vi "Version3.0.vi"() -> ()   [LabVIEW 2012]
uses:
  <vilib>/Instr/_visa.llb/VISA Configure Serial Port (Instr).vi
  Function_Set/Debug/Function_Set.dll
panel:
  in  "选项卡控件":enum32{"Note", "AVT CCD", "Vacuum REC", "..."}(tab)
  in  "Double:":dbl
  in  "String:":string
  in  "Other:":string
  in  "Save This Shot":bool
  out "Shots:":i32
  in  "Save This Notes":bool
  in  "Other Notes:":string
  out "Shot's situation:":string
  out "Shots: 2":i32
  out "Notes:":string
  in  "查询":bool
  in  "Options":u16(ring) caption="Choose File:"
  in  "Initial Folder Path:":path
  in  "Your Own:":u16(ring) items=["2, 10000, 3, 1", "2, 10000, 4, 1"]
  in  "FrameStartTriggerMode":T1(ring)
  in  "AcquisitionMode":T2(ring)
  in  "ExposureMode":T3(ring)
  in  "AVT SDK Demon":bool
  out "CCD ID":string
  out "ExposureMode":string
  out "ExposureValue":u32
  out "AcquisitionMode":string
  out "FrameStartTriggerMode":string
  in  "ExposureValue":u32
  in  "CameraStart":bool
  in  "CameraStop":bool
  in  "CameraSet":bool
  in  "CameraGet":bool
  in  "CameraSetAll":bool
  in  "path to JPEG file":path caption="Path of the Pic"
  out "new picture":picture caption="Pic"
  in  "端口选择":refnum<visa-resource-name>="COM1"
  in  "baud rate":u32=9600
  in  "data bits":u16=8
  in  "stop bits":u16(ring)=10 items=["1.0"=10, "1.5"=15, "2.0"=20]
  in  "flow control":u16(ring) items=["None"=0, "XON/XOFF"=1, "RTS/CTS"=2, "DTR/DSR"=4]
  in  "timeout":u32=10
  in  "RS485地址":string="12"
  in  "读取间隔(s)":dbl=1.0 caption="Delay Time (s)"
  in  "数据文件夹":string="data"
  in  "记录说明":string="test"
  out "数据路径":path
  in  "parity (0:none)":enum16{"None", "Odd", "Even", "Mark", "Space"}(ring)
  in  "记录所有读取数据?":bool
  out "已记录数据点":u32 caption="recorded number"
  in  "stop":bool
  out "电离规图表":dbl(graph)
  out "电阻规图表":dbl(graph)
  out "已读取数据点":i32
  out "预定耗时":dbl
  out "实际耗时":dbl
  in  "临界压强(Pa)":dbl=8.0
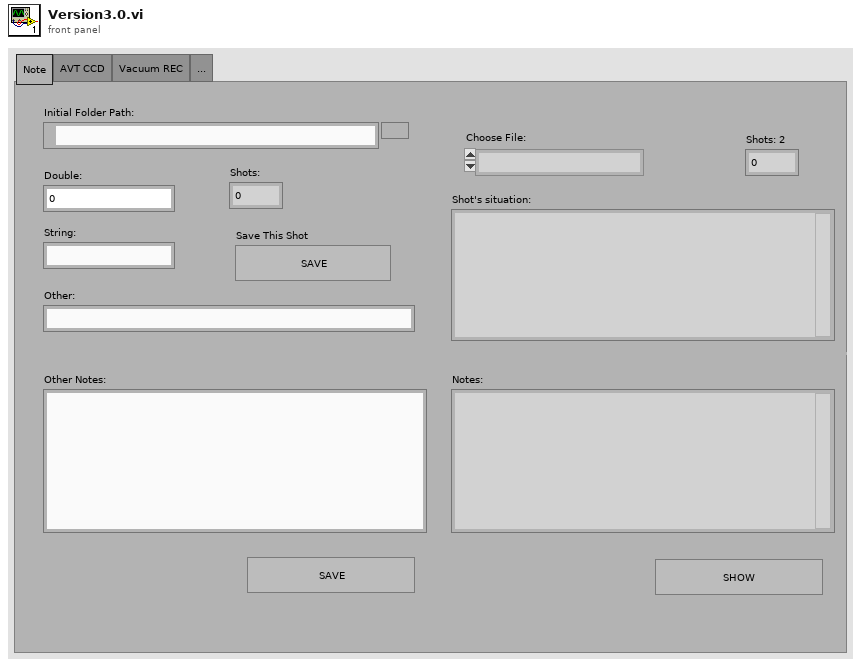
[diagram p1: front panel]
types:
  T1 = enum16{"默认", "Freerun", "SyncIn1", "SyncIn2", "FixedRate", "Software"}
  T2 = enum16{"默认", "Continuous", "SingleFrame", "MultiFrame", "Recorder"}
  T3 = enum16{"默认", "Manual", "Auto", "AutoOnce", "External"}
  T4 = cluster{"Resister":dbl, "Ionization":dbl, "time":string, "Ionization":dbl, "Ionization":dbl, u32, i32}
  T5 = enum32{"Record", "Instrument 1", "Instrument 2", "..."}
  T6 = enum16{"open", "replace", "create", "open or create", "replace or create", "replace or create with confirmation"}
  T7 = typedef "imagedata.ctl" = cluster{"image type":i32, "image depth":i32, "image":u8[], "mask":u8[], "colors":u32[], "Rectangle":cluster{"left":i16, "top":i16, "right":i16, "bottom":i16}}
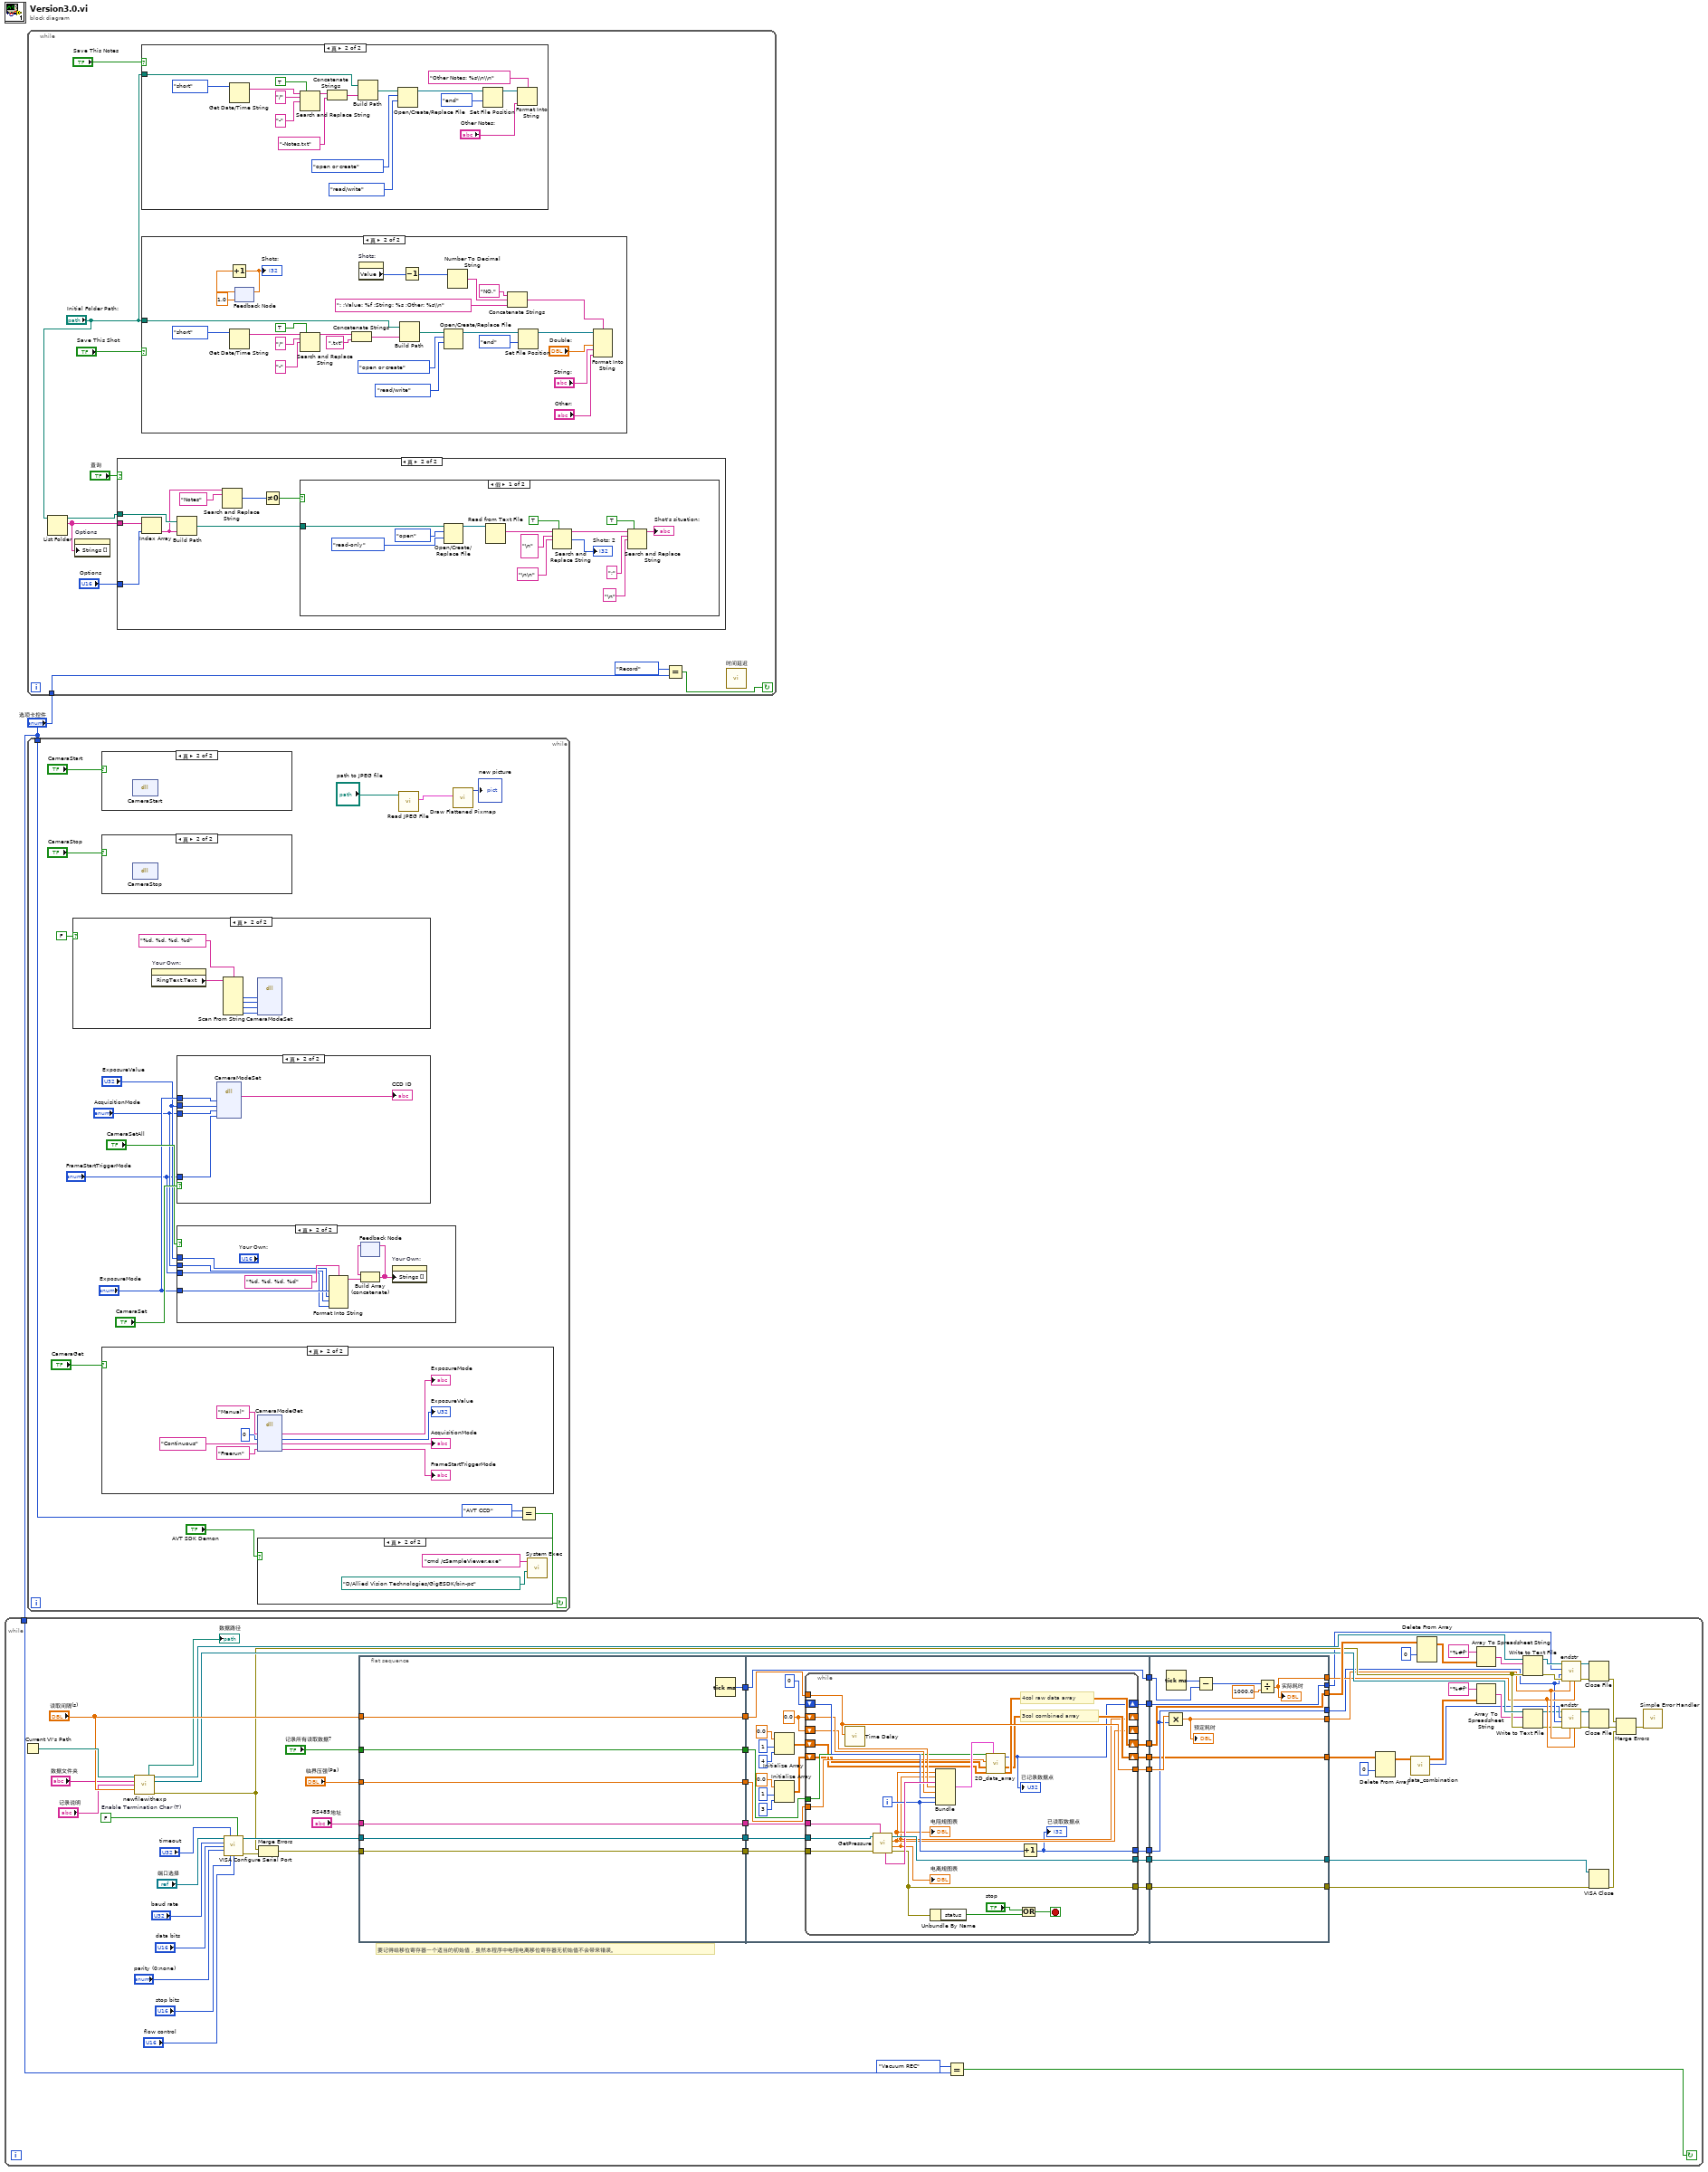
[diagram p0: block diagram]
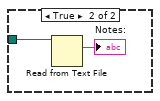
[diagram p10: hidden frame]
diagram:
  n1 = while {
    tunnel: "选项卡控件" -> [w3]
    stop <- w4 continue-if-true
    w54 = FALSE  # Enable Termination Char (T)
    # "要记得给移位寄存器一个适当的初始值，虽然本程序中电阻电离移位寄存器无初始值不会带来错误。"
    n2 = Current VI's Path() -> (path=w46:path)
    n3 = call "newfilewithexp.vi"("路径"=w46, "数据文件夹"="数据文件夹", "记录说明"="记录说明", "读取间隔(s)"="读取间隔(s)") -> ("数据路径"=→"数据路径":path, "refnum out for 4column"=w25:refnum<file>, "refnum out for 3column"=w23:refnum<file>, "error out"=w22:errorcluster)  [unwired: 1 in, 7 out]
    n4 = call-poly "VISA Configure Serial Port"("VISA resource name"="端口选择", "timeout (10sec)"="timeout", "Enable Termination\nChar (T)"=w54, "baud rate (9600)"="baud rate", "data bits (8)"="data bits", "parity (0:none)"="parity (0:none)", "stop bits (10: 1 bit)"="stop bits", "flow control (0:none)"="flow control") -> ("VISA resource name out"=w51:refnum<visa-resource-name>, "error out"=w26:errorcluster)  [unwired: 1 in, 5 out]
    n5 = Merge Errors(w22, w26) -> (w34:errorcluster)
    n6 = flat-sequence {
      tunnel: "RS485地址" -> [w74]
      tunnel: "读取间隔(s)" -> [w75]
      tunnel: "记录所有读取数据?" -> [w76]
      tunnel: w34 -> [w77]
      tunnel: w51 -> [w78]
      tunnel: [w78] -> w71
      tunnel: [w77] -> w70
      tunnel: [w76] -> w69
      tunnel: [w75] -> w68
      tunnel: [w74] -> w67
      tunnel: [w73] -> w66
      tunnel: "临界压强(Pa)" -> [w72]
      tunnel: [w72] -> w65
      tunnel: [w100] -> w64
      tunnel: [w79] -> w63
      tunnel: w71 -> [w102]
      tunnel: w70 -> [w101]
      tunnel: w69 -> [w98]
      tunnel: w68 -> [w97]
      tunnel: w67 -> [w96]
      tunnel: [w95] -> w62
      tunnel: w66 -> [w95]
      tunnel: [w94] -> w61
      tunnel: [w93] -> w60
      tunnel: w65 -> [w92]
      tunnel: [w91] -> w59
      tunnel: [w85] -> w58
      tunnel: [w80] -> w57
      tunnel: [w139] -> w49
      tunnel: [w140] -> w50
      tunnel: w64 -> [w140]
      tunnel: w63 -> [w139]
      tunnel: w62 -> [w137]
      tunnel: w61 -> [w131]
      tunnel: w60 -> [w134]
      tunnel: w59 -> [w132]
      tunnel: w58 -> [w133]
      tunnel: [w133] -> w39
      tunnel: [w132] -> w18
      tunnel: [w131] -> w17
      tunnel: [w130] -> w20
      tunnel: [w129] -> w19
      tunnel: w57 -> [w128]
      tunnel: [w128] -> w33
      frame #0 {
        n7 = Tick Count (ms)() -> (millisecond timer value=w73:u32)
      }
      frame #1 {
        w90 = 0.0 ("Ionization")
        n8 = Initialize Array(0.0 ("element"), 1 ("dimension size"), 4 ("dimension size")) -> (w88:dbl[][])
        n9 = Initialize Array(0.0 ("element"), 1 ("dimension size"), 3 ("dimension size")) -> (w81:dbl[][])
        n10 = while {
          tunnel: w102 -> [w127]
          tunnel: w101 -> [w126]
          tunnel: w96 -> [w123]
          tunnel: [w109] -> w100
          tunnel: [w124] -> w79
          shift-right: [w110] -> w91
          shift-left: u32 0 -> [w120]
          shift-right: [w104] -> _
          shift-left: w90 -> [w119]
          tunnel: w97 -> [w125]
          tunnel: w98 -> [w116]
          tunnel: [w103] -> w94
          tunnel: [w125] -> w93
          shift-right: [w105] -> _
          shift-left: w90 -> [w118]
          tunnel: w92 -> [w115]
          shift-right: [w113] -> w85
          shift-left: w88 -> [w114]
          shift-right: [w111] -> w80
          shift-left: w81 -> [w112]
          i -> [w121]
          stop <- w106 stop-if-true
          # "4col raw data array"
          # "3col combined array"
          n11 = call "Time Delay"("Delay Time (s)"=w125) -> ()  [unwired: 1 in, 10 out]
          n12 = call "GetPressure.vi"("Address of RS485"=w123, "error in (no error)"=w126, "VISA resource name"=w127) -> ("error out"=w109:errorcluster, "Ionization"=w104:dbl, "Resister"=w105:dbl, "VISA resource name out"=w124:refnum<visa-resource-name>, "time"=w122:string)  [unwired: 1 in, 3 out]
          "电阻规图表" <- w105
          "电离规图表" <- w104
          n13 = Unbundle By Name(w109) -> ("status"=w107:bool)
          n14 = Bundle("Resister"=w105, "Ionization"=w104, "time"=w122, "Ionization"=w118, "Ionization"=w119, w120, w121) -> (w117:T4)  [unwired: 1 out]
          n15 = call "2D_data_array.vi"("input cluster"=w117, "input 4column array"=w114, "input combined 3column array"=w112, "critical pressure"=w115, "record all data points?"=w116) -> ("output 4column array"=w113:dbl[][], "output combined 3column array"=w111:dbl[][], "recorded number out"=w110:u32)  [unwired: 4 out]
          "已记录数据点" <- w110
          n16 = Or(x="stop", y=w107) -> (x .or. y?=w106:bool)
          n17 = Increment(x=w121) -> (x+1=w103:i32)
          "已读取数据点" <- w103
        }
      }
      frame #2 {
        n18 = Multiply(x=w134, y=w131) -> (x*y=w130:dbl)
        "预定耗时" <- w130
        n19 = Tick Count (ms)() -> (millisecond timer value=w138:u32)
        n20 = Subtract(x=w138, y=w137) -> (x-y=w136:u32)
        n21 = Divide(x=w136, y=1000.0) -> (x/y=w129:dbl)
        "实际耗时" <- w129
      }
    }
    n22 = Equal?(x=enum32{"Note", "AVT CCD", "Vacuum REC", "..."}."Vacuum REC", y=w3) -> (x = y?=w4:bool)
    n23 = Delete From Array(array=w33, index (row)=0) -> (array with subset deleted=w30:dbl[][])  [unwired: 2 in, 1 out]
    n24 = call "data_combination.vi"("input combined data array"=w30) -> ("recorded combined data number"=w16:i32, "output combined data array"=w27:dbl[][])  [unwired: 9 out]
    n25 = Delete From Array(array=w39, index (row)=0) -> (array with subset deleted=w40:dbl[][])  [unwired: 2 in, 1 out]
    n26 = Array To Spreadsheet String(array=w40, 3:"%#f" ("format string")) -> (spreadsheet string=w24:string)  [unwired: 1 out]
    n27 = Array To Spreadsheet String(array=w27, 3:"%#f" ("format string")) -> (spreadsheet string=w21:string)  [unwired: 1 out]
    n28 = Write to Text File(file (use dialog)=w25, text=w24, error in=w22) -> (refnum out=w36:refnum<file>, error out=w35:errorcluster)  [unwired: 2 out]
    n29 = Write to Text File(file (use dialog)=w23, text=w21, error in=w22) -> (refnum out=w15:refnum<file>, error out=w14:errorcluster)  [unwired: 2 out]
    n30 = call "endstr.vi"("实际耗时"=w19, "预定耗时"=w20, "error in"=w35, "已读取数据点"=w17, "已记录数据点"=w18, "refnum in"=w36) -> ("error out"=w38:errorcluster, "refnum out"=w37:refnum<file>)  [unwired: 4 out]
    n31 = call "endstr.vi"("实际耗时"=w19, "预定耗时"=w20, "error in"=w14, "已读取数据点"=w17, "已记录数据点"=w16, "refnum in"=w15) -> ("error out"=w28:errorcluster, "refnum out"=w29:refnum<file>)  [unwired: 4 out]
    n32 = Close File(refnum=w37, error in=w38) -> (error out=w10:errorcluster)  [unwired: 1 out]
    n33 = Close File(refnum=w29, error in=w28) -> (error out=w11:errorcluster)  [unwired: 1 out]
    n34 = VISA Close(VISA resource name=w49, error in (no error)=w50) -> (error out=w12:errorcluster)
    n35 = Merge Errors(w10, w11, w12) -> (w13:errorcluster)
    n36 = call <vilib>:"Simple Error Handler.vi"("error in (no error)"=w13) -> ()  [unwired: 1 in, 8 out]
  }
  n37 = while {
    tunnel: "选项卡控件" -> [w143]
    stop <- w144 continue-if-true
    n38 = List Folder(path="Initial Folder Path:") -> (path out=w147:path, filenames=w145:string[])  [unwired: 3 in, 2 out]
    n39 = property on="Options" class="Ring (严格)"("Strings []"=w145) -> ()  [unwired: 2 in, 2 out]
    n40 = case shown="真" "查询" {
      tunnel: w145 -> [_ w158]
      tunnel: "Options" -> [_ w157]
      tunnel: w147 -> [_ w156]
      frame False {
      }
      frame True {
        n41 = Index Array(array=w158, index=w157) -> (element=w155:string)
        n42 = Build Path(base path=w156, name or relative path=w155) -> (appended path=w151:path)
        n43 = Search and Replace String(input string=w155, search string="Notes" ("搜索字符串")) -> (number of replacements=w153:i32)  [unwired: 6 in, 3 out]
        n44 = Not Equal To 0?(x=w153) -> (x != 0?=w152:bool)
        n45 = case shown="假" w152 {
          tunnel: w151 -> [w172 w174]
          frame False {
            n46 = Open/Create/Replace File(file path (use dialog)=w172, operation (0:open)=T6."open" ("操作(0:open)"), access (0:read/write)=enum16{"read/write", "read-only", "write-only"}."read-only" ("权限(0:read/write)")) -> (refnum out=w169:refnum<file>)  [unwired: 3 in, 2 out]
            n47 = Read from Text File(file (use dialog)=w169) -> (text=w165:string)  [unwired: 3 in, 3 out]
            n48 = Search and Replace String(replace all?=TRUE ("替换全部？(F)"), input string=w165, search string="\n" ("搜索字符串"), replace string="\n\n" ("替换字符串(\"\")")) -> (result string=w162:string, number of replacements=→"Shots: 2":i32)  [unwired: 4 in, 2 out]
            n49 = Search and Replace String(replace all?=TRUE ("替换全部？(F)"), input string=w162, search string=";" ("搜索字符串"), replace string="\n" ("替换字符串(\"\")")) -> (result string=→"Shot's situation:":string)  [unwired: 4 in, 3 out]
          }
          frame True {
            n50 = Read from Text File(file (use dialog)=w174) -> (text=→"Notes:":string)  [unwired: 3 in, 3 out]
          }
        }
      }
    }
    n51 = case shown="真" "Save This Notes" {
      tunnel: "Initial Folder Path:" -> [_ w175]
      frame False {
      }
      frame True {
        n52 = Get Date/Time String(date format (0)=enum16{"short", "long", "abbreviated"}."short" ("日期格式(0)")) -> (date string=w187:string)  [unwired: 2 in, 1 out]
        n53 = Search and Replace String(replace all?=TRUE ("替换全部？(F)"), input string=w187, search string="/" ("搜索字符串"), replace string="-" ("替换字符串(\"\")")) -> (result string=w178:string)  [unwired: 4 in, 3 out]
        n54 = Concatenate Strings(w178, "-Notes.txt" ("字符串")) -> (w176:string)
        n55 = Build Path(base path=w175, name or relative path=w176) -> (appended path=w188:path)
        n56 = Open/Create/Replace File(file path (use dialog)=w188, operation (0:open)=T6."open or create" ("操作(0:open)"), access (0:read/write)=enum16{"read/write", "read-only", "write-only"}."read/write" ("权限(0:read/write)")) -> (refnum out=w181:refnum<file>)  [unwired: 3 in, 2 out]
        n57 = Set File Position(refnum=w181, from (0:start)=enum16{"start", "end", "current"}."end" ("自（0:起始）")) -> (refnum out=w180:refnum<file>)  [unwired: 2 in, 1 out]
        n58 = Format Into String(format string="Other Notes: %s\\n\\n" ("格式字符串"), initial string=w180, "Other Notes:") -> ()  [unwired: 1 in, 2 out]
      }
    }
    n59 = case shown="真" "Save This Shot" {
      tunnel: "Initial Folder Path:" -> [_ w198]
      frame False {
      }
      frame True {
        n60 = Get Date/Time String(date format (0)=enum16{"short", "long", "abbreviated"}."short" ("日期格式(0)")) -> (date string=w212:string)  [unwired: 2 in, 1 out]
        n61 = feedback #1(1.0 ("x")) -> (w201:dbl)
        n62 = Increment(x=w201) -> (x+1=w199:dbl)
        "Shots:" <- w199
        n63 = feedback-in #1(w199) -> ()
        n64 = Search and Replace String(replace all?=TRUE ("替换全部？(F)"), input string=w212, search string="/" ("搜索字符串"), replace string="-" ("替换字符串(\"\")")) -> (result string=w209:string)  [unwired: 4 in, 3 out]
        n65 = Concatenate Strings(w209, ".txt" ("字符串")) -> (w214:string)
        n66 = property on="Shots:" class="DigNum (严格)"() -> ("Value"=w193:i32)  [unwired: 2 in, 2 out]
        n67 = Build Path(base path=w198, name or relative path=w214) -> (appended path=w215:path)
        n68 = Decrement(x=w193) -> (x-1=w192:i32)
        n69 = Open/Create/Replace File(file path (use dialog)=w215, operation (0:open)=T6."open or create" ("操作(0:open)"), access (0:read/write)=enum16{"read/write", "read-only", "write-only"}."read/write" ("权限(0:read/write)")) -> (refnum out=w203:refnum<file>)  [unwired: 3 in, 2 out]
        n70 = Number To Decimal String(number=w192) -> (decimal integer string=w197:string)  [unwired: 1 in]
        n71 = Concatenate Strings("NO." ("字符串"), w197, ": ;Value: %f ;String: %s ;Other: %s\\n" ("格式字符串")) -> (w194:string)
        n72 = Set File Position(refnum=w203, from (0:start)=enum16{"start", "end", "current"}."end" ("自（0:起始）")) -> (refnum out=w202:refnum<file>)  [unwired: 2 in, 1 out]
        n73 = Format Into String(format string=w194, initial string=w202, "Double:", "String:", "Other:") -> ()  [unwired: 1 in, 2 out]
      }
    }
    n74 = Equal?(x=T5."Record", y=w143) -> (x = y?=w144:bool)
    n75 = call "时间延迟"() -> ()  [unwired: 11 in, 1 out]
  }
  n76 = while {
    tunnel: "选项卡控件" -> [w220]
    stop <- w221 continue-if-true
    n77 = case shown="真" FALSE {
      frame False {
      }
      frame True {
        n78 = property on="Your Own:" class="Ring (严格)"() -> ("RingText.Text"=w236:string)  [unwired: 2 in, 2 out]
        n79 = Scan From String(format string="%d, %d, %d, %d" ("格式字符串"), input string=w236) -> (output 1=w238:i32, output 2=w239:i32, output 3=w240:i32, output 4=w241:i32)  [unwired: 6 in, 3 out]
        n80 = dll-call lib="F:/Kun's Test/Function_Set/Debug/Function_Set.dll" fn="CameraModeSet"("EM"=w238, "EV"=w239, "AM"=w240, "FSTM"=w241) -> ()  [unwired: 8 in, 2 out]
      }
    }
    n81 = case shown="真" "CameraStart" {
      frame False {
      }
      frame True {
        n82 = dll-call lib="F:/Kun's Test/Function_Set/Debug/Function_Set.dll" fn="CameraStart"() -> ()  [unwired: 4 in, 2 out]
      }
    }
    n83 = case shown="真" "CameraStop" {
      frame False {
      }
      frame True {
        n84 = dll-call lib="F:/Kun's Test/Function_Set/Debug/Function_Set.dll" fn="CameraStop"() -> ()  [unwired: 4 in, 2 out]
      }
    }
    n85 = case shown="真" "CameraGet" {
      frame False {
      }
      frame True {
        n86 = dll-call lib="F:/Kun's Test/Function_Set/Debug/Function_Set.dll" fn="CameraModeGet"("ExposureMode"="Manual", "ExposureValue"=u32 0, "AcquisitionMode"="Continuous", "FrameStartTriggerMode"="Freerun") -> ("ExposureMode"=→"ExposureMode":string, "ExposureValue"=→"ExposureValue":u32, "AcquisitionMode"=→"AcquisitionMode":string, "FrameStartTriggerMode"=→"FrameStartTriggerMode":string)  [unwired: 4 in, 2 out]
      }
    }
    n87 = case shown="真" "CameraSet" {
      tunnel: "ExposureValue" -> [_ w261]
      tunnel: "ExposureMode" -> [_ w260]
      tunnel: "AcquisitionMode" -> [_ w259]
      tunnel: "FrameStartTriggerMode" -> [_ w258]
      frame False {
      }
      frame True {
        n88 = dll-call lib="F:/Kun's Test/Function_Set/Debug/Function_Set.dll" fn="CameraModeSet"("EM"=w260, "EV"=w261, "AM"=w259, "FSTM"=w258) -> ("返回类型"=→"CCD ID":string)  [unwired: 7 in, 2 out]
      }
    }
    n89 = case shown="真" "CameraSetAll" {
      tunnel: "ExposureMode" -> [_ w245]
      tunnel: "ExposureValue" -> [_ w244]
      tunnel: "AcquisitionMode" -> [_ w243]
      tunnel: "FrameStartTriggerMode" -> [_ w242]
      frame False {
      }
      frame True {
        n90 = Format Into String(format string="%d, %d, %d, %d" ("格式字符串"), w245, w244, w243, w242) -> (resulting string=w248:string)  [unwired: 2 in, 1 out]
        n91 = feedback #2() -> (w247:string[])  [unwired: 1 in]
        n92 = Build Array (concatenate)(w247, w248) -> (w246:string[])
        n93 = feedback-in #2(w246) -> ()
        n94 = property on="Your Own:" class="Ring (严格)"("Strings []"=w246) -> ()  [unwired: 2 in, 2 out]
      }
    }
    n95 = case shown="真" "AVT SDK Demon" {
      frame False {
      }
      frame True {
        n96 = call <vilib>:"System Exec.vi"("working directory"=path "D:/Allied Vision Technologies/GigESDK/bin-pc", "command line"="cmd /cSampleViewer.exe") -> ()  [unwired: 6 in, 4 out]
      }
    }
    n97 = call <vilib>:"Read JPEG File.vi"("path to JPEG file"="path to JPEG file") -> ("image data"=w222:T7)  [unwired: 8 in, 2 out]
    n98 = call <vilib>:"Draw Flattened Pixmap.vi"("image data"=w222) -> ("new picture"=→"new picture":picture)  [unwired: 8 in]
    n99 = Equal?(x=enum32{"Note", "AVT CCD", "Vacuum REC", "..."}."AVT CCD", y=w220) -> (x = y?=w221:bool)
  }
